vi "Encoders.vi"() -> ()   [LabVIEW 2013]
uses:
  <vilib>/Rock Robotics/SystemInterfaces/DIO/FPGA_DIOChannel.ctl
  <vilib>/Rock Robotics/WPI/Encoder/WPI_EncoderType.ctl
  <vilib>/Rock Robotics/WPI/Counter/WPI_CounterDigitalInputToDigitalSource.vi
panel:
  out "Encoder Rate (distance/sec)":dbl
  out "Encoder Distance":dbl
  in  "stop":bool
  in  "Reset Encoder?":bool
  out "Encoder Alarm Status":string
  out "Encoder Direction":string
  in  "Number Samples to Average":u8=1 min=1 max=128
  in  "Invert Direction":bool
  in  "Decoding Type":T1=enum."4x"
  in  "DistancePerCount":dbl=1.0
  in  "B Channel":T2=enum."DIO 2"
  in  "A Channel":T2
  in  "Minimum Rate":dbl=20.0
  in  "State Control":enum16{"Open", "Run", "End"}(ring)
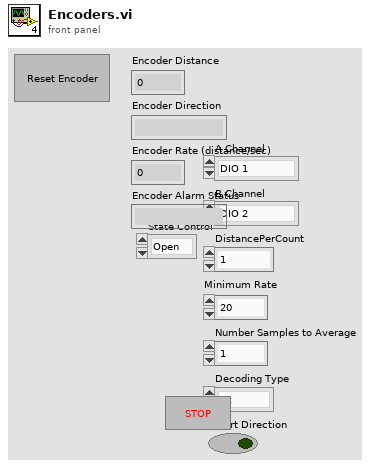
[diagram p1: front panel]
types:
  T1 = typedef "WPI_EncoderType.ctl" = enum16{"1x", "2x", "4x"}
  T2 = typedef "FPGA_DIOChannel.ctl" = enum8{"DIO 1", "DIO 2", "DIO 3", "DIO 4", "DIO 5", "DIO 6", "DIO 7", "DIO 8", "DIO 9", "DIO 10", "DIO 11", "DIO 12", "DIO 13", "DIO 14", "Invalid"}
  T3 = typedef "WPI_DigitalInputDevRef.ctl" = cluster{"DevStatus":errorcluster, "DIO Channel":T2, "Digital Module":T4}
  T4 = typedef "FPGA_TypedefDigitalModule.ctl" = enum16{"Digital Module 1", "Digital Module 2"}
  T5 = typedef "FPGA_CounterEncoderSourceConvertionLVSourceType.ctl" = cluster{"DevStatus":errorcluster, "AnalogTriggerMode?":bool, "DigitalMode":cluster{"Digital Module":T4, "DIO Channel":T6}, "AnalogTriggerMode":cluster{"AnalogTriggerIndex":T7, "OutputType":T8}}
  T6 = typedef "FPGA_DIODigitalSourceChannel.ctl" = enum8{"DIO 1", "DIO 2", "DIO 3", "DIO 4", "DIO 5", "DIO 6", "DIO 7", "DIO 8", "DIO 9", "DIO 10", "DIO 11", "DIO 12", "DIO 13", "DIO 14", "Disabled"}
  T7 = typedef "FPGA_AnalogTriggerIndex.ctl" = enum8{"Trig 0", "Trig 1", "Trig 2", "Trig 3", "Trig 4", "Trig 5", "Trig 6", "Trig 7", "Invalid"}
  T8 = typedef "FPGA_AnalogTriggerOutType.ctl" = enum16{"InWindow", "TriggerState", "Rising", "Falling"}
  T9 = typedef "WPI_EncoderDevRef.ctl" = cluster{"DevStatus":errorcluster, "EncoderIndex":T10, "CounterIndex":T11, "DistancePerCount":dbl, "Decoding Type":T1}
  T10 = typedef "FPGA_EncoderIdx.ctl" = enum8{"Enc 0", "Enc 1", "Enc 2", "Enc 3", "Invalid"}
  T11 = typedef "FPGA_CounterCtrSystemIndex.ctl" = enum8{"Ctr 0", "Ctr 1", "Ctr 2", "Ctr 3", "Ctr 4", "Ctr 5", "Ctr 6", "Ctr 7", "Invalid"}
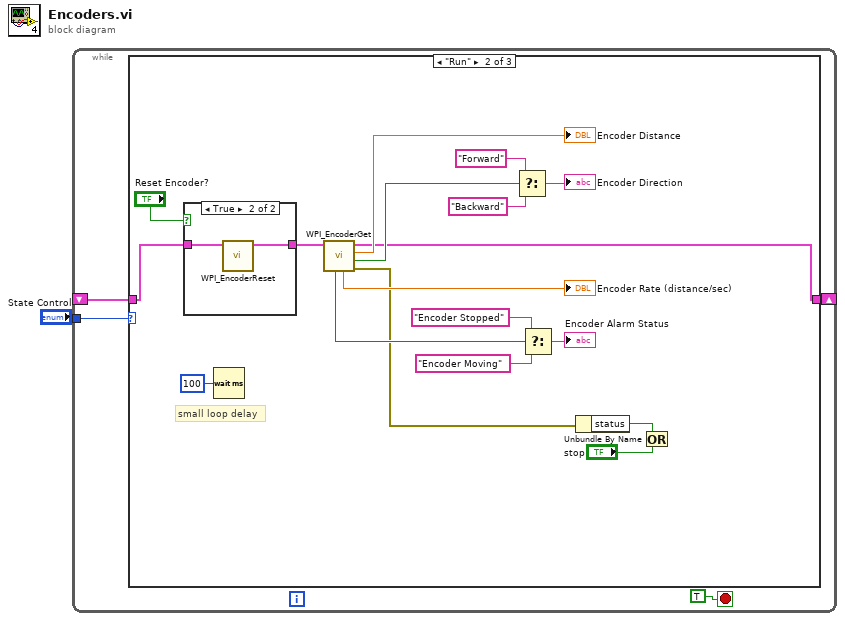
[diagram p0: block diagram]
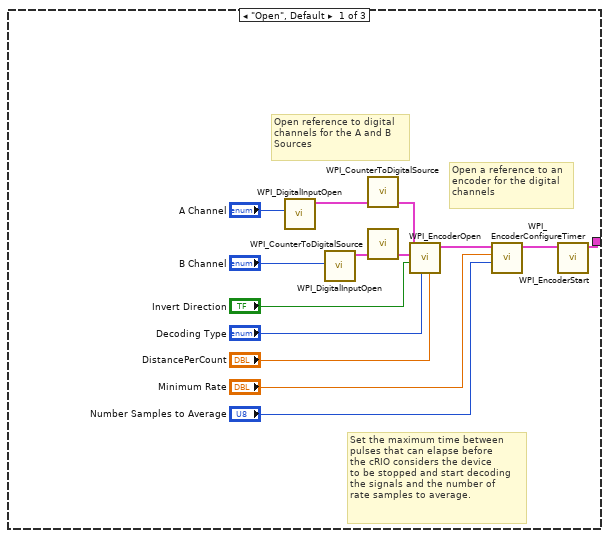
[diagram p2: hidden frame]
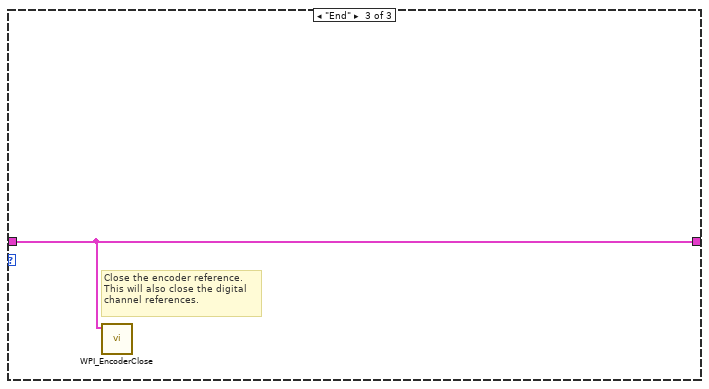
[diagram p4: hidden frame]
diagram:
  n1 = while {
    tunnel: "State Control" -> [w5]
    shift-right: [w3] -> _
    shift-left: _ -> [w2]
    stop <- TRUE stop-if-true
    n2 = case shown="\"Run\"" w5 {
      tunnel: [w6 w21 w41] -> w3
      tunnel: w2 -> [_ w20 w41]
      frame "Open", Default {
        # "Set the maximum time between\npulses that can elapse before \nthe cRIO considers the device \nto be stopped and start decoding\nthe signals and the number of\nrate samples to average."
        # "Open a reference to an\nencoder for the digital \nchannels"
        # "Open reference to digital \nchannels for the A and B\nSources"
        n3 = call <vilib>:"WPI_DigitalInputOpen.vi"("DIO Channel"="A Channel") -> ("DigitalInputDevRef"=w17:T3)  [unwired: 2 in, 8 out]
        n4 = call <vilib>:"WPI_DigitalInputOpen.vi"("DIO Channel"="B Channel") -> ("DigitalInputDevRef"=w18:T3)  [unwired: 2 in, 8 out]
        n5 = call-poly <vilib>:"WPI_CounterToDigitalSource.vi"("DigitalInputDevRef"=w17) -> ("Digital Source"=w16:T5)  [unwired: 6 out]
        n6 = call-poly <vilib>:"WPI_CounterToDigitalSource.vi"("DigitalInputDevRef"=w18) -> ("Digital Source"=w19:T5)  [unwired: 6 out]
        n7 = call <vilib>:"WPI_EncoderOpen.vi"("DistancePerCount"="DistancePerCount", "Decoding Type"="Decoding Type", "Invert Direction (False)"="Invert Direction", "BSource"=w19, "ASource"=w16) -> ("EncoderDevRef"=w9:T9)  [unwired: 3 in, 3 out]
        n8 = call <vilib>:"WPI_EncoderConfigureTimer.vi"("Number Samples to Average"="Number Samples to Average", "Minimum Rate"="Minimum Rate", "EncoderDevRef"=w9) -> ("EncoderDevRef"=w10:T9)  [unwired: 1 in, 7 out]
        n9 = call <vilib>:"WPI_EncoderStart.vi"("EncoderDevRef"=w10) -> ("EncoderDevRef"=w6:T9)  [unwired: 1 in, 9 out]
      }
      frame "Run" {
        # "small loop delay"
        n10 = case shown="True" "Reset Encoder?" {
          tunnel: w20 -> [w38 w39]
          tunnel: [w38 w40] -> w34
          frame False {
          }
          frame True {
            n11 = call <vilib>:"WPI_EncoderReset.vi"("EncoderDevRef"=w39) -> ("EncoderDevRef"=w40:T9)  [unwired: 1 in, 9 out]
          }
        }
        n12 = Wait (ms)(milliseconds to wait=u32 100) -> ()  [unwired: 1 out]
        n13 = call <vilib>:"WPI_EncoderGet.vi"("EncoderDevRef"=w34) -> ("error out"=w28:errorcluster, "Direction"=w33:bool, "Distance"=→"Encoder Distance":dbl, "EncoderDevRef"=w21:T9, "Rate"=→"Encoder Rate (distance/sec)":dbl, "Stopped"=w32:bool)  [unwired: 1 in, 4 out]
        n14 = Select(t="Forward", s=w33, f="Backward") -> (s? t:f=→"Encoder Direction":string)
        n15 = Select(t="Encoder Stopped", s=w32, f="Encoder Moving") -> (s? t:f=→"Encoder Alarm Status":string)
        n16 = Unbundle By Name(w28) -> ("status"=w26:bool)
        n17 = Or(x=w26, y="stop") -> ()  [unwired: 1 out]
      }
      frame "End" {
        # "Close the encoder reference.\nThis will also close the digital \nchannel references."
        n18 = call <vilib>:"WPI_EncoderClose.vi"("EncoderDevRef"=w41) -> ()  [unwired: 2 in, 9 out]
      }
    }
  }
